vi "Initialize.vi"(8 "error in (no error)":errorcluster, 10 "Internal?":bool, 11 "Julabo FP-50 Settings":T2={"VISA resource name"="", "Simulated?"=FALSE, "Pump Power"=2} {"Pump Power" min=0 max=8 step=1}) -> (0 "error out":errorcluster, 2 "Connection Error":bool, 3 "Julabo FP-50 Settings":T2={"VISA resource name"="", "Simulated?"=FALSE, "Pump Power"=2} {"Pump Power" min=0 max=8 step=1})   [LabVIEW 2021, in "Julabo Type FP-50 TCU.lvlib"]
uses:
  Julabo Type FP-50 TCU.lvlib
  Julabo FP-50 Settings.ctl
  Third Party Drivers/Julabo Type 1/JULABO DeviceDriver/JULABO DeviceDriver.lvlib
panel:
  in  "Serial Configuration":T1={"Baud Rate"=4800, "Parity"=0, "Data Bits"=8, "Stop Bits"=10, "Flow Control"=2} {"Baud Rate" items=["300"=300, "600"=600, "1200"=1200, "2400"=2400, "4800"=4800, "9600"=9600, "19200"=19200]; "Parity" items=["None", "Odd", "Even", "Mark", "Space"]; "Data Bits" items=["7"=7, "7"=8]; "Stop Bits" items=["1.0"=10, "1.5"=15, "2.0"=20]; "Flow Control" items=["None", "XON/XOFF", "RTS/CTS", "XON/XOFF & RTS/CTS", "DTR/DSR", "XON/XOFF & DTR/DSR"]}
  out "error out 2":errorcluster
  in  "Reset / Default (T: Both)":bool=TRUE
  in  "ID Query? (T: Yes)":bool=TRUE
  in  "RS485-Address (128: RS232)":u32=128
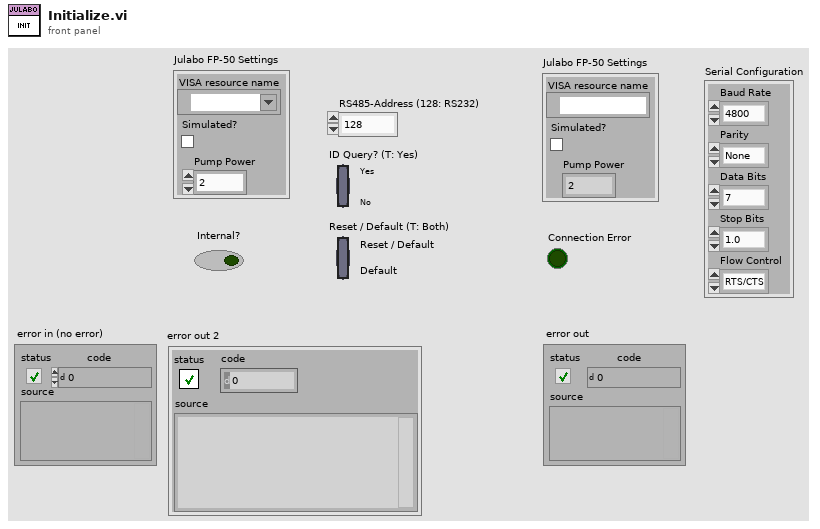
[diagram p1: front panel]
types:
  T1 = cluster{"Baud Rate":u32, "Parity":u16, "Data Bits":u16, "Stop Bits":u16, "Flow Control":u16}
  T2 = typedef "Julabo Type FP-50 TCU.lvlib/Julabo FP-50 Settings.ctl" = cluster{"VISA resource name":refnum<visa-resource-name>, "Simulated?":bool, "Pump Power":i32}
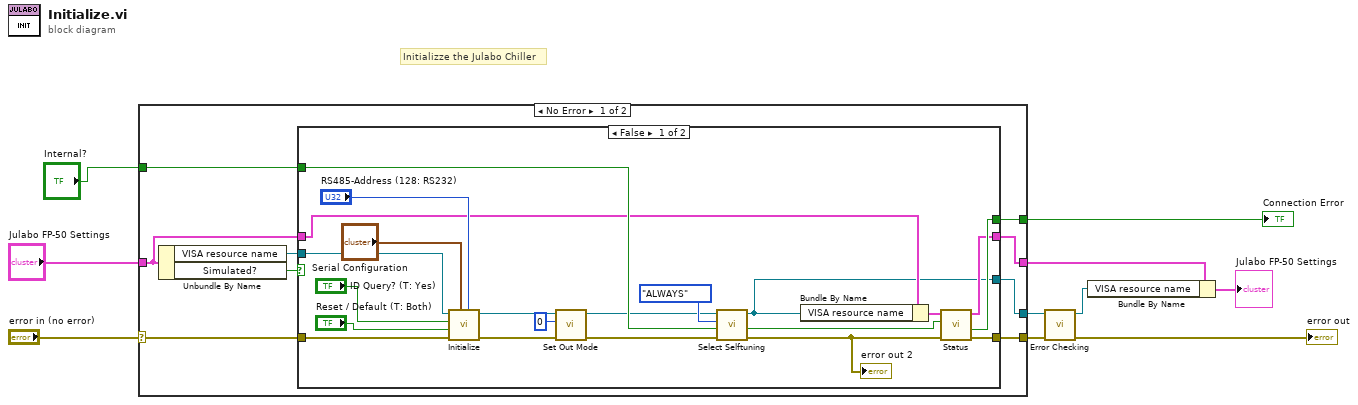
[diagram p0: block diagram]
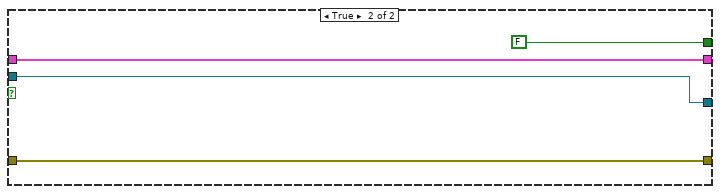
[diagram p2: hidden frame]
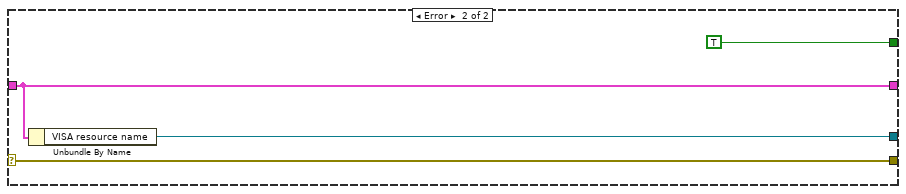
[diagram p3: hidden frame]
diagram:
  # "Initializze the Julabo Chiller"
  n1 = case shown="No Error" "error in (no error)" {
    selector: "error in (no error)" -> [w19 w47]
    tunnel: "Julabo FP-50 Settings" -> [w13 w44]
    tunnel: [w18 w47] -> w8
    tunnel: [w16 w46] -> w9
    tunnel: [w14 TRUE] -> w4
    tunnel: [w12 w44] -> w3
    tunnel: "Internal?" -> [w11 _]
    frame No Error {
      n2 = Unbundle By Name(w13) -> ("VISA resource name"=w17:refnum<visa-resource-name>, "Simulated?"=w15:bool)
      n3 = case shown="False" w15 {
        tunnel: w19 -> [w30 w43]
        tunnel: [w36 w43] -> w18
        tunnel: [w20 w42] -> w16
        tunnel: w17 -> [w31 w42]
        tunnel: [w38 FALSE] -> w14
        tunnel: w13 -> [w28 w40]
        tunnel: [w37 w40] -> w12
        tunnel: w11 -> [w29 _]
        frame False {
          n4 = call "Initialize.vi"("RS485-Address (128: RS232)"="RS485-Address (128: RS232)", "Serial Configuration"="Serial Configuration", "error in (no error)"=w30, "Reset / Default (T: Both)"="Reset / Default (T: Both)", "ID Query? (T: Yes)"="ID Query? (T: Yes)", "VISA resource name"=w31) -> ("error out"=w23:errorcluster, "VISA resource name out"=w25:refnum<visa-resource-name>)  [unwired: 4 in]
          n5 = call "Set Out Mode.vi"("error in (no error)"=w23, "Out Mode 1"=u8 0, "VISA resource name"=w25) -> ("error out"=w22:errorcluster, "VISA resource name out"=w24:refnum<visa-resource-name>)  [unwired: 7 in]
          n6 = call "Select Selftuning.vi"("error in (no error)"=w22, "Selftuning (0: OFF)"=enum16{"OFF", "ONCE", "ALWAYS"}."ALWAYS", "VISA resource name"=w24) -> ("error out"=w26:errorcluster, "VISA resource name out"=w20:refnum<visa-resource-name>)  [unwired: 7 in]
          "error out 2" <- w26
          n7 = Bundle By Name(cluster=w28, "VISA resource name"=w20) -> (w39:T2)
          n8 = call "Status.vi"("error in (no error)"=w26, "Internal?"=w29, "Julabo FP-50 Settings In"=w39) -> ("error out"=w36:errorcluster, "Connection Error"=w38:bool, "Julabo FP-50 Settings Out"=w37:T2)  [unwired: 3 in, 3 out]
        }
        frame True {
        }
      }
    }
    frame Error {
      n9 = Unbundle By Name(w44) -> ("VISA resource name"=w46:refnum<visa-resource-name>)
    }
  }
  "Connection Error" <- w4
  n10 = call "Error Checking.vi"("error in (no error)"=w8, "VISA resource name"=w9) -> ("error out"=→"error out":errorcluster, "VISA resource name"=w6:refnum<visa-resource-name>)  [unwired: 7 in, 1 out]
  n11 = Bundle By Name(cluster=w3, "VISA resource name"=w6) -> (→"Julabo FP-50 Settings":T2)
